vi "Test 2 Parse Response When Measuring Voltage.vi"(8 "error in (no error)":errorcluster, 11 "Test Case In":refnum<class "Driver Test.lvclass">) -> (0 "error out":errorcluster, 3 "Test Case Out":refnum<class "Driver Test.lvclass">)   [LabVIEW 2020, in "Driver Test.lvclass"]
uses:
  Driver Test.lvclass
  C:/Program Files (x86)/National Instruments/LabVIEW 2020/vi.lib/Astemes/LUnit/Test Case.lvclass
  <vilib>/Astemes/LUnit/Test Case.lvclass/Test Case.ctl
  e83b171a-c1d6-4db8-9d64-19d6ae92fd3f.vi
  <vilib>/Astemes/LUnit/Append Pass Result.vi
  <vilib>/Astemes/LUnit/Append Fail Result.vi
  <vilib>/Astemes/LUnit/Describe Comparison.vi
  <vilib>/Astemes/LUnit/Compare Variants.vi
  <vilib>/Astemes/LUnit/Variant to string.vi
  Mock Serial/Mock Serial.lvclass
  C:/git/astemes-lmock/sandbox/Examples/Serial/Serial.lvclass/Serial.lvclass
  <vilib>/Utility/Data Type/Get Type Information.vi
  <vilib>/Utility/LVClass/Get LV Class Name.vi
  Driver/Driver.lvclass
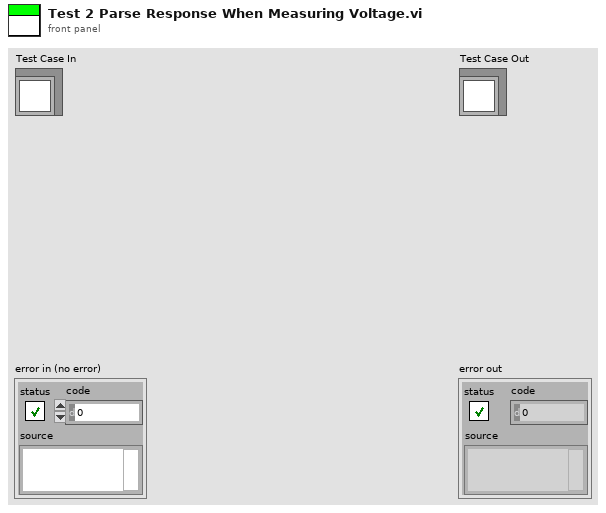
[diagram p1: front panel]
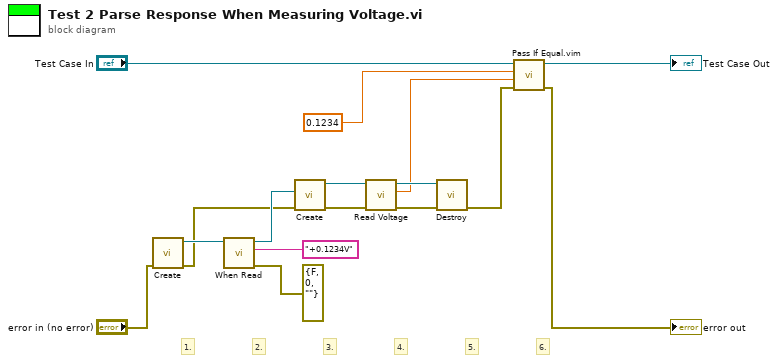
[diagram p0: block diagram]
diagram:
  # "6."
  # "5."
  # "4."
  # "3."
  # "2."
  # "1."
  n1 = call "Create.vi"("error in (no error)"="error in (no error)") -> ("error out"=w3:errorcluster, "Mock Class Generator out"=w5:refnum<class "Mock Serial.lvclass">)  [unwired: 9 in]
  n2 = call "When Read.vi"("error out"=errorcluster {"status"=FALSE, "code"=0, "source"=""}, "read buffer"="+0.1234V" ("write buffer"), "Serial in"=w5) -> ("Serial out"=w8:refnum<class "Mock Serial.lvclass">)  [unwired: 8 in]
  n3 = call "Create.vi"("error in (no error)"=w3, "Serial"=w8) -> ("error out"=w13:errorcluster, "Driver"=w11:refnum<class "Driver.lvclass">)  [unwired: 8 in]
  n4 = call "Read Voltage.vi"("error in (no error)"=w13, "Driver In"=w11) -> ("error out"=w12:errorcluster, "Voltage"=w1:dbl, "Driver Out"=w10:refnum<class "Driver.lvclass">)  [unwired: 7 in]
  n5 = call "Destroy.vi"("error in (no error)"=w12, "Driver"=w10) -> ("error out"=w7:errorcluster)  [unwired: 9 in]
  n6 = call "Pass If Equal.vim"("error in (no error)"=w7, "Actual"=w1, "Expected"=0.1234, "LUnit Test Case In"="Test Case In") -> ("error out"=→"error out":errorcluster, "LUnit Test Case Out"=→"Test Case Out":refnum<class "Driver Test.lvclass">)  [unwired: 6 in]
